vi "Add Tests.vi"(8 "error in (no error)":errorcluster, 10 "Tests":string[](array[string]), 11 "Result Model by Reference In":refnum<class "Result Model.lvclass">) -> (0 "error out":errorcluster)   [LabVIEW 2020, in "Result Model.lvclass"]
uses:
  Result Model/Result Model.lvclass
  Result Model/Result Model.lvclass/Result Model.ctl
  00fc22c9-78c8-43fd-a5ea-589dbb8ac889.vi
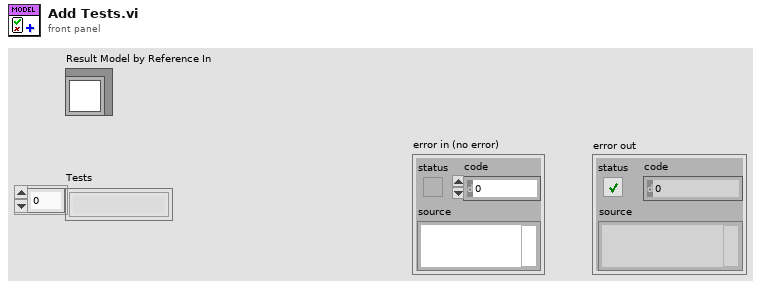
[diagram p1: front panel]
types:
  T1 = typedef "Result.lvlib/Status.ctl" = enum16{"", "Passed", "Failed", "Error", "Skipped", "Setup Error", "Broken", "Teardown Error"}
  T2 = typedef "Result.lvlib/Type.ctl" = enum16{"Test Case", "Test Suite", "Test Run", "Pass", "Fail", "Skip", "Pass if", "Fail if", "Pass if Error", "Fail if Error", "Pass if Equal", "Fail if Equal"}
  T3 = cluster{"Tests":string[], "Run Queue":string[], "Test Statuses":map{string, T1}, "Execution Time":map{string, dbl}, "Assertions":map{string, cluster{"Result Type":T2, "Status":T1, "Description":string, "Data":cluster{"Expected":variant, "Actual":variant, "Delta":variant}}[]}}
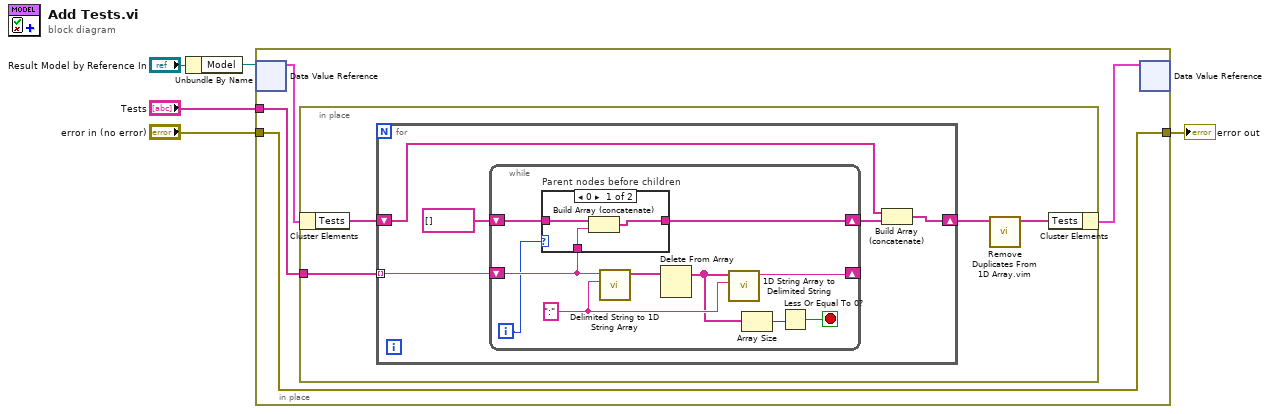
[diagram p0: block diagram]
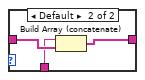
[diagram p2: hidden frame]
diagram:
  n1 = Unbundle By Name("Result Model by Reference In") -> ("Model"=w5:refnum<data-value>)
  n2 = in-place {
    in-place-border: "error in (no error)" -> [w9]
    in-place-border: [w9] -> w1
    in-place-border: "Tests" -> [w6]
    n3 = in-place-dvr #1(w5) -> (w7:T3)  [unwired: 1 out]
    n4 = in-place {
      in-place-border: w6 -> [w13]
      n5 = in-place-cluster #2(w7) -> ("Tests"=w12:string[])
      n6 = for {
        tunnel: w13 -> [w18] mode=indexing
        shift-right: [w15] -> w11
        shift-left: w12 -> [w14]
        n7 = while {
          shift-right: [w25] -> _
          shift-left: w18 -> [w21]
          shift-right: [w20] -> w17
          shift-left: string[] [] -> [w22]
          i -> [w19]
          stop <- w23 stop-if-true
          w27 = ":" ("delimiter")
          n8 = case "Parent nodes before children" shown="0" w19 {
            tunnel: w22 -> [w31 w34]
            tunnel: w21 -> [w30 w33]
            tunnel: [w29 w32] -> w20
            frame 0 {
              n9 = Build Array (concatenate)(w31, w30) -> (w29:string[])
            }
            frame Default {
              n10 = Build Array (concatenate)(w33, w34) -> (w32:string[])
            }
          }
          n11 = call <vilib>:"Delimited String to 1D String Array.vi"("delimiter"=w27, "delimited string"=w21) -> ("string array"=w28:string[])  [unwired: 9 in]
          n12 = Delete From Array(array=w28) -> (array with subset deleted=w26:string[])  [unwired: 2 in, 1 out]
          n13 = call <vilib>:"1D String Array to Delimited String.vi"("delimiter"=w27, "string array"=w26) -> ("delimited string"=w25:string)  [unwired: 9 in]
          n14 = Array Size(array=w26) -> (size(s)=w24:i32)
          n15 = Less Or Equal To 0?(x=w24) -> (x <= 0?=w23:bool)
        }
        n16 = Build Array (concatenate)(w14, w17) -> (w15:string[])
      }
      n17 = call "Remove Duplicates From 1D Array.vim"("array"=w11) -> ("array with duplicates removed"=w10:string[])  [unwired: 10 in]
      n18 = in-place-cluster #2("Tests"=w10) -> (w8:T3)
    }
    n19 = in-place-dvr #1(w8) -> ()  [unwired: 2 out]
  }
  "error out" <- w1
